vi "Init Effect UI.vi"(11 "Effect Info":T1) -> ()   [LabVIEW 2019, in "Effect Unit.lvclass"]
uses:
  Effect Unit.lvclass
  Effect Info.ctl
  Plugin Interfaces/Effect Interface/Effect Interface.lvlibp/Effect Interface Class/Effect Interface.lvclass
  Packed Libraries/Messaging.lvlibp/Message Cluster.ctl
  Packed Libraries/Messaging.lvlibp
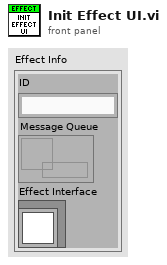
[diagram p1: front panel]
types:
  T1 = typedef "Effect Unit.lvclass/Effect Info.ctl" = cluster{"ID":string, "Message Queue":refnum<queue>, "Effect Interface":refnum<class "Effect Interface.lvclass">}
  T2 = typedef "Audio Processing.lvlibp/Value Cluster.ctl" = cluster{"Value":dbl, "Properties":T3}
  T3 = typedef "Audio Processing.lvlibp/Value Properties.ctl" = cluster{"Lower":dbl, "Upper":dbl, "Default":dbl, "Increment":dbl}
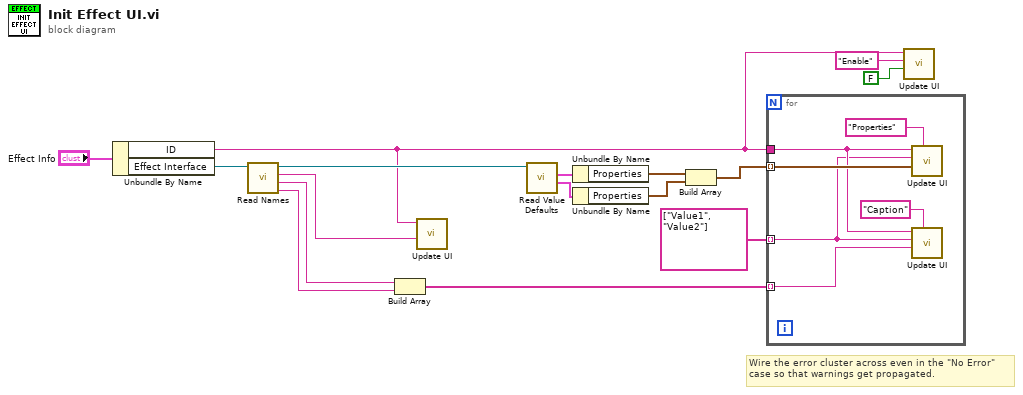
[diagram p0: block diagram]
diagram:
  # "Wire the error cluster across even in the \"No Error\"\ncase so that warnings get propagated."
  n1 = Unbundle By Name("Effect Info") -> ("ID"=w3:string, "Effect Interface"=w13:refnum<class "Effect Interface.lvclass">)
  n2 = call "Read Names.vi"("Effect Interface in"=w13) -> ("Value2 Name"=w6:string, "Value1 Name"=w7:string, "Effect Name"=w4:string, "Effect Interface out"=w12:refnum<class "Effect Interface.lvclass">)  [unwired: 7 in]
  n3 = Build Array(w7, w6) -> (w5:string[])
  n4 = call "Update UI.vi"("Data"=w4, "ID"=w3) -> ()  [unwired: 9 in, 1 out]
  n5 = call "Read Value Defaults.vi"("Effect Interface in"=w12) -> ("Value2"=w9:T2, "Value1"=w11:T2)  [unwired: 8 in, 1 out]
  n6 = Unbundle By Name(w11) -> ("Properties"=w10:T3)
  n7 = Unbundle By Name(w9) -> ("Properties"=w8:T3)
  n8 = Build Array(w10, w8) -> (w15:T3[])
  n9 = for {
    tunnel: w3 -> [w20]
    tunnel: w15 -> [w22] mode=indexing
    tunnel: string[] ["Value1", "Value2"] -> [w18] mode=indexing
    tunnel: w5 -> [w17] mode=indexing
    n10 = call "Update UI.vi"("Message (Value Change)"="Properties", "Data"=w22, "Target"=w18, "ID"=w20) -> ()  [unwired: 7 in, 1 out]
    n11 = call "Update UI.vi"("Message (Value Change)"="Caption", "Data"=w17, "Target"=w18, "ID"=w20) -> ()  [unwired: 7 in, 1 out]
  }
  n12 = call "Update UI.vi"("Data"=FALSE, "Target"="Enable", "ID"=w3) -> ()  [unwired: 8 in, 1 out]
